vi "TCPWriteWithSize.vi"(8 "error in (no error)":errorcluster, 10 "Command String":string, 11 "Connection In":refnum<k5>) -> (0 "error out":errorcluster, 3 "Connection out":refnum<k5>)   [LabVIEW 2015]
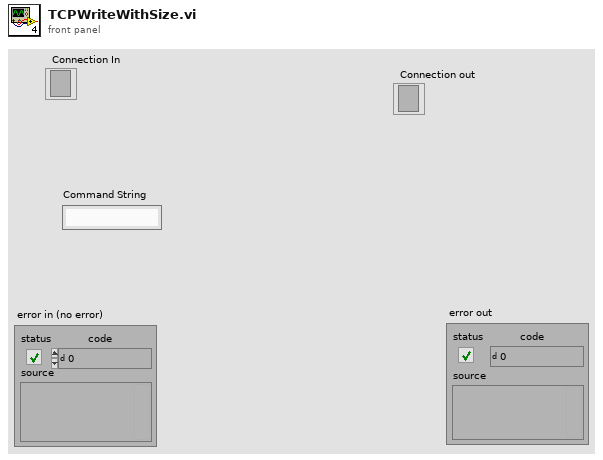
[diagram p1: front panel]
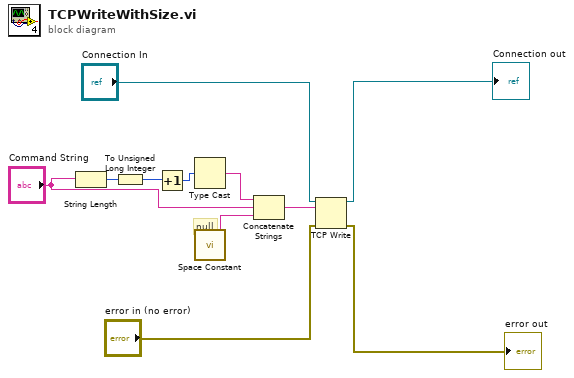
[diagram p0: block diagram]
diagram:
  # "null"
  n1 = String Length(string="Command String") -> (length=w10:i32)
  n2 = To Unsigned Long Integer(number=w10) -> (unsigned 32bit integer=w9:u32)
  n3 = Increment(x=w9) -> (x+1=w8:u32)
  n4 = Type Cast(x=w8) -> (*(type *) &x=w11:string)  [unwired: 1 in]
  n5 = call <vilib>:"Space Constant.vi"() -> ("String"=w6:string)
  n6 = Concatenate Strings(w11, "Command String", w6) -> (w5:string)
  n7 = TCP Write(connection ID="Connection In", data in=w5, error in (no error)="error in (no error)") -> (connection ID out=→"Connection out":refnum<k5>, error out=→"error out":errorcluster)  [unwired: 1 in, 1 out]
